vi "Calibrate.vi"() -> ()   [LabVIEW 2013]
uses:
  <vilib>/Rock Robotics/WPI/RobotDrive/WPI_RobotDriveMecanumDrive_Cartesian.vi
panel:
  out "Start Time":u32
  in  "Motor Speed":dbl
  in  "Max Stopped Period":dbl
  in  "Initiate Calibration":bool
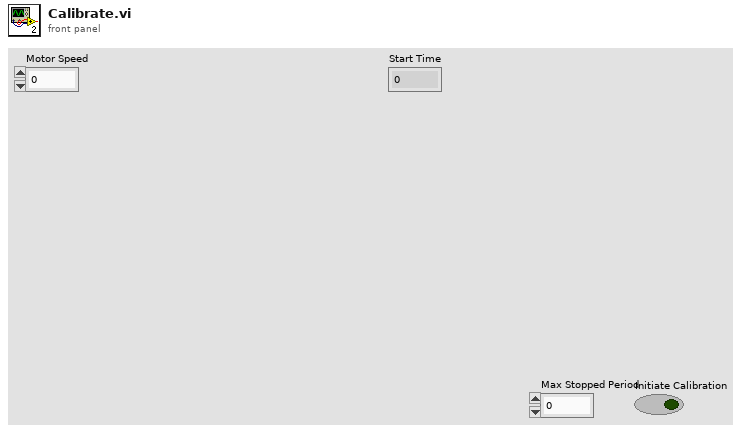
[diagram p1: front panel]
types:
  T1 = typedef "WPI_CounterDevRef.ctl" = cluster{"DevStatus":errorcluster, "CntIndex":T2}
  T2 = typedef "FPGA_CounterCtrSystemIndex.ctl" = enum8{"Ctr 0", "Ctr 1", "Ctr 2", "Ctr 3", "Ctr 4", "Ctr 5", "Ctr 6", "Ctr 7", "Invalid"}
  T3 = typedef "WPI_RobotDriveDevRef.ctl" = cluster{"DevStatus":errorcluster, "Motors[]":T4[], "Square Inputs":bool, "Max Output":dbl, "Isochronous":bool}
  T4 = typedef "WPI_MotorControlDeviceRef.ctl" = cluster{"DeviceStatus":errorcluster, "Type":enum16{"PWM", "CAN"}, "PWM":cluster{"Digital Module":T5, "PWM Channel":T6, "DeadBand":T7}, "CAN":cluster{"Device Number":u8, "Control Mode":T8, "Semaphore":T9, "Max Vout":dbl}, "Invert":bool, "TransformRef":T10, "InvTransformRef":T10}
  T5 = typedef "FPGA_TypedefDigitalModule.ctl" = enum16{"Digital Module 1", "Digital Module 2"}
  T6 = typedef "FPGA_DIOPWMChannel.ctl" = enum8{"PWM 1", "PWM 2", "PWM 3", "PWM 4", "PWM 5", "PWM 6", "PWM 7", "PWM 8", "PWM 9", "PWM 10", "Invalid"}
  T7 = typedef "WPI_PWMDeadband.ctl" = cluster{"Name":string, "maxPositivePwm":i32, "minPositivePwm":i32, "centerPwm":i32, "maxNegativePwm":i32, "minNegativePwm":i32, "angularRange":u16}
  T8 = typedef "WPI_CANJaguar_ControlMode.ctl" = enum8{"Percent VBus", "Current", "Speed", "Position", "Voltage"}
  T9 = typedef "Semaphore RefNum" = refnum<k1>
  T10 = typedef "WPI_PWMTransform_ConPane.ctl" = refnum<vi>
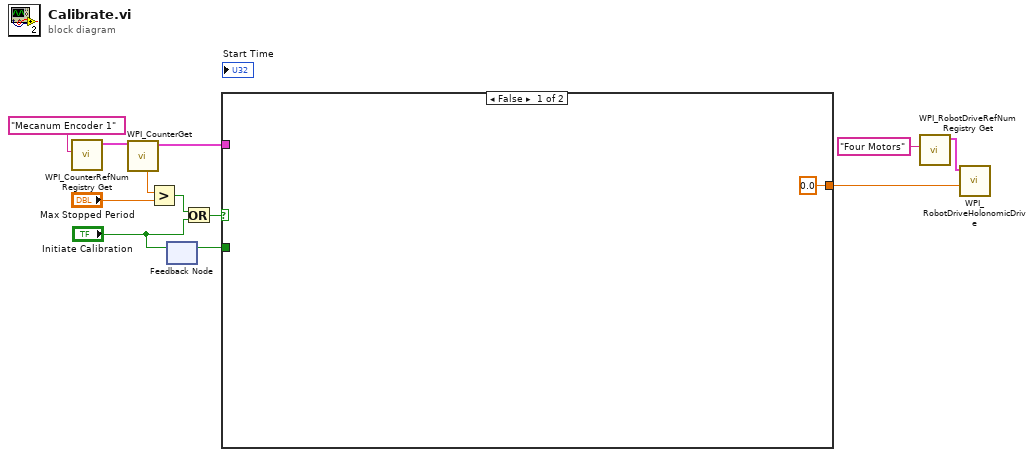
[diagram p0: block diagram]
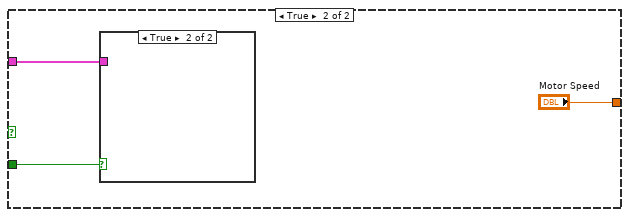
[diagram p2: hidden frame]
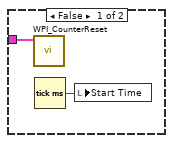
[diagram p3: hidden frame]
diagram:
  n1 = call <vilib>:"WPI_CounterRefNum Registry Get.vi"("refnum name"="Mecanum Encoder 1") -> ("CounterDevRef"=w11:T1)  [unwired: 9 in, 1 out]
  n2 = call <vilib>:"WPI_CounterGet.vi"("CounterDevRef in"=w11) -> ("CounterDevRef out"=w1:T1, "Period (sec)"=w9:dbl)  [unwired: 5 in, 4 out]
  n3 = Greater?(x=w9, y="Max Stopped Period") -> (0:w8:bool)
  n4 = feedback-in #1("Initiate Calibration") -> ()
  n5 = feedback #1() -> (w5:bool)  [unwired: 1 in]
  n6 = Or(x=w8, y="Initiate Calibration") -> (x .or. y?=w7:bool)
  n7 = case shown="False" w7 {
    tunnel: w5 -> [_ w16]
    tunnel: [0.0 ("Motor Speed") "Motor Speed"] -> w2
    tunnel: w1 -> [_ w14]
    frame False {
    }
    frame True {
      n8 = case shown="True" w16 {
        tunnel: w14 -> [w18 _]
        frame False {
          n9 = call <vilib>:"WPI_CounterReset.vi"("CounterDevRef in"=w18) -> ()  [unwired: 9 in, 2 out]
          n10 = Tick Count (ms)() -> (millisecond timer value=w17:u32)
          n11 = local write "Start Time"(w17) -> ()
        }
        frame True {
        }
      }
    }
  }
  n12 = call <vilib>:"WPI_RobotDriveRefNum Registry Get.vi"("refnum name"="Four Motors") -> ("RobotDriveDevRef"=w4:T3)  [unwired: 1 in, 9 out]
  n13 = call-poly <vilib>:"WPI_RobotDriveHolonomicDrive.vi"("Y"=w2, "RobotDriveDevRef"=w4) -> ()  [unwired: 7 in, 3 out]
